vi "Store New VI for Category List.vi"(6 "Help Text":string, 8 "error in (no error)":errorcluster, 9 "String":string, 10 "VI Refnum":refnum<vi>, 11 "Configuration in":refnum<class "Configuration.lvclass">) -> (0 "error out":errorcluster, 3 "Configuration out":refnum<class "Configuration.lvclass">)   [LabVIEW 2016, in "Configuration.lvlib" / "Configuration.lvclass"]
uses:
  <userlib>/Configuration Dialog Actor/Configuration.lvclass
  <userlib>/Configuration Dialog Actor/Configuration.lvclass/Configuration.ctl
  <userlib>/Configuration Dialog Actor/Methods/Data Retrieved by Lookup Table.ctl
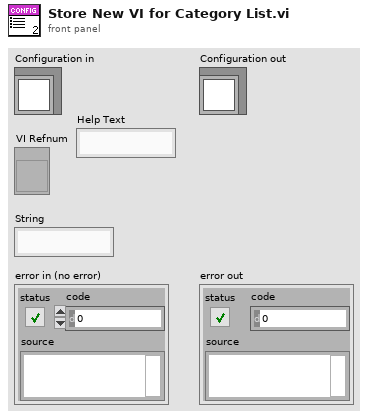
[diagram p1: front panel]
types:
  T1 = typedef "Configuration.lvlib/Configuration.lvclass/Data Retrieved by Lookup Table.ctl" = cluster{"VI Refnum":refnum<vi>, "Help Text":string}
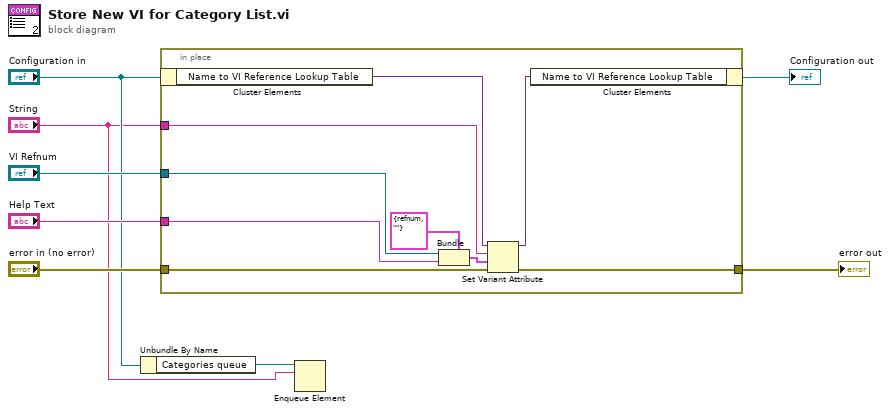
[diagram p0: block diagram]
diagram:
  n1 = Unbundle By Name("Configuration in") -> ("Categories queue"=w2:refnum<queue>)
  n2 = in-place {
    in-place-border: "VI Refnum" -> [w12]
    in-place-border: "String" -> [w15]
    in-place-border: "error in (no error)" -> [w14]
    in-place-border: [w13] -> w7
    in-place-border: "Help Text" -> [w11]
    n3 = in-place-cluster #1("Configuration in") -> ("Name to VI Reference Lookup Table"=w17:variant)
    n4 = Bundle(cluster=T1 {"VI Refnum"=refnum, "Help Text"=""} ("output cluster"), "VI Refnum"=w12, "Help Text"=w11) -> (w10:T1)
    n5 = Set Variant Attribute(Variant=w17, name=w15, value=w10, error in=w14) -> (Variant out=w16:variant, error out=w13:errorcluster)  [unwired: 1 out]
    n6 = in-place-cluster #1("Name to VI Reference Lookup Table"=w16) -> (→"Configuration out":refnum<class "Configuration.lvclass">)
  }
  "error out" <- w7
  n7 = Enqueue Element(queue=w2, element="String") -> ()  [unwired: 2 in, 3 out]
